vi "Save_GSF_Data.vi"(8 "error in":errorcluster, 9 "time format string (%c)":string="Data\\%d_%B_%y\\%H_%M_%S_", 10 "Save":bool, 11 "GSF_Data":dbl[][](array[numeric])) -> (0 "error out":errorcluster)   [LabVIEW 2021]
uses:
  <vilib>/Utility/file.llb/Write Delimited Spreadsheet (DBL).vi
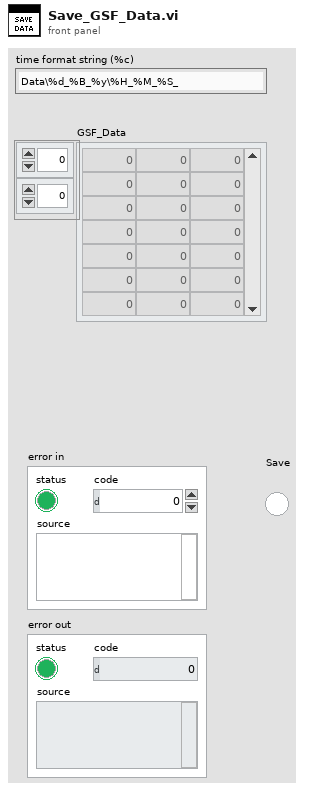
[diagram p1: front panel]
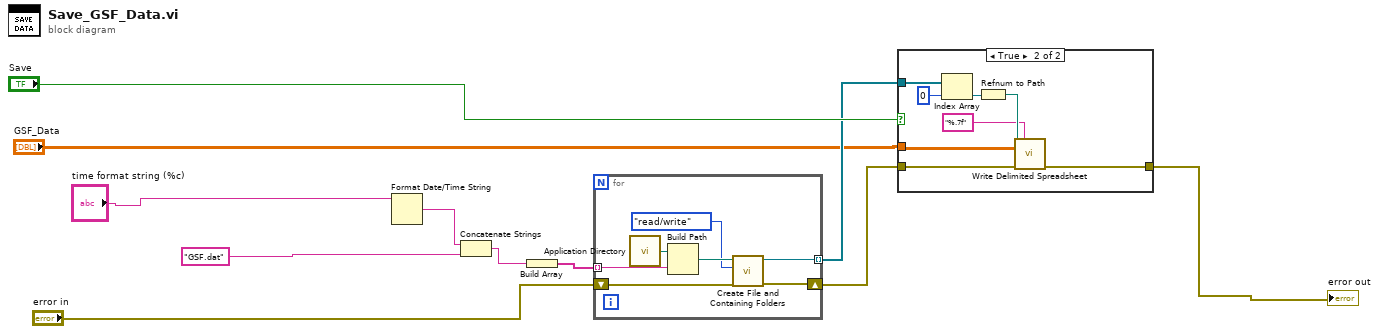
[diagram p0: block diagram]
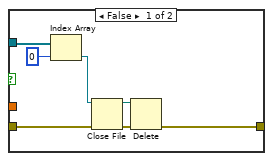
[diagram p2: hidden frame]
diagram:
  n1 = Format Date/Time String(time format string (%c)="time format string (%c)") -> (date/time string=w4:string)  [unwired: 2 in]
  n2 = Concatenate Strings(w4, "GSF.dat") -> (w11:string)
  n3 = Build Array(w11) -> (w10:string[])
  n4 = for {
    tunnel: [w12] -> w6 mode=indexing
    tunnel: w10 -> [w15] mode=indexing
    shift-right: [w13] -> w7
    shift-left: "error in" -> [w14]
    n5 = call <vilib>:"Application Directory.vi"() -> ("Application Directory"=w17:path)
    n6 = Build Path(base path=w17, name or relative path=w15) -> (appended path=w18:path)
    n7 = call <vilib>:"Create File and Containing Folders.vi"("error in (no error)"=w14, "access"=enum16{"read/write", "read-only", "write-only"}."read/write", "file path"=w18) -> ("error out"=w13:errorcluster, "refnum out"=w12:refnum<file>)  [unwired: 7 in]
  }
  n8 = case shown="True" "Save" {
    tunnel: w6 -> [w24 w32]
    tunnel: "GSF_Data" -> [_ w31]
    tunnel: w7 -> [w20 w30]
    tunnel: [w23 w29] -> w3
    frame False {
      n9 = Index Array(array=w24, index=0) -> (element=w21:refnum<file>)
      n10 = Close File(refnum=w21, error in=w20) -> (path=w22:path, error out=w19:errorcluster)
      n11 = Delete(path (use dialog)=w22, error in=w19) -> (error out=w23:errorcluster)  [unwired: 3 in, 2 out]
    }
    frame True {
      n12 = Index Array(array=w32, index=0) -> (element=w28:refnum<file>)
      n13 = Refnum to Path(1:w28) -> (0:w27:path)
      n14 = call-poly <vilib>:"Write Delimited Spreadsheet.vi"("file path (dialog if empty)"=w27, "format (%.3f)"="%.7f", "2D data"=w31, "error in (no error)"=w30) -> ("error out"=w29:errorcluster)  [unwired: 10 in, 1 out]
    }
  }
  "error out" <- w3
